vi "Lesson1 - Producer-Consumer Architecture and Queues.vi"() -> ()   [LabVIEW 2013]
uses:
  <vilib>/measure/NI_MABase.lvlib
panel:
  out "Waveform Graph":dbl[](graph)
  in  "Stop Button":bool
  out "Numeric 2":i32
  out "Numeric":i32
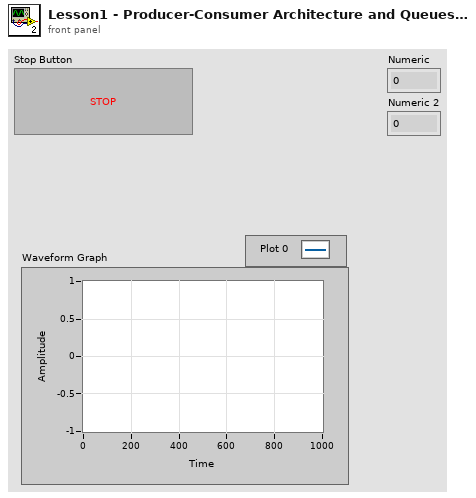
[diagram p1: front panel]
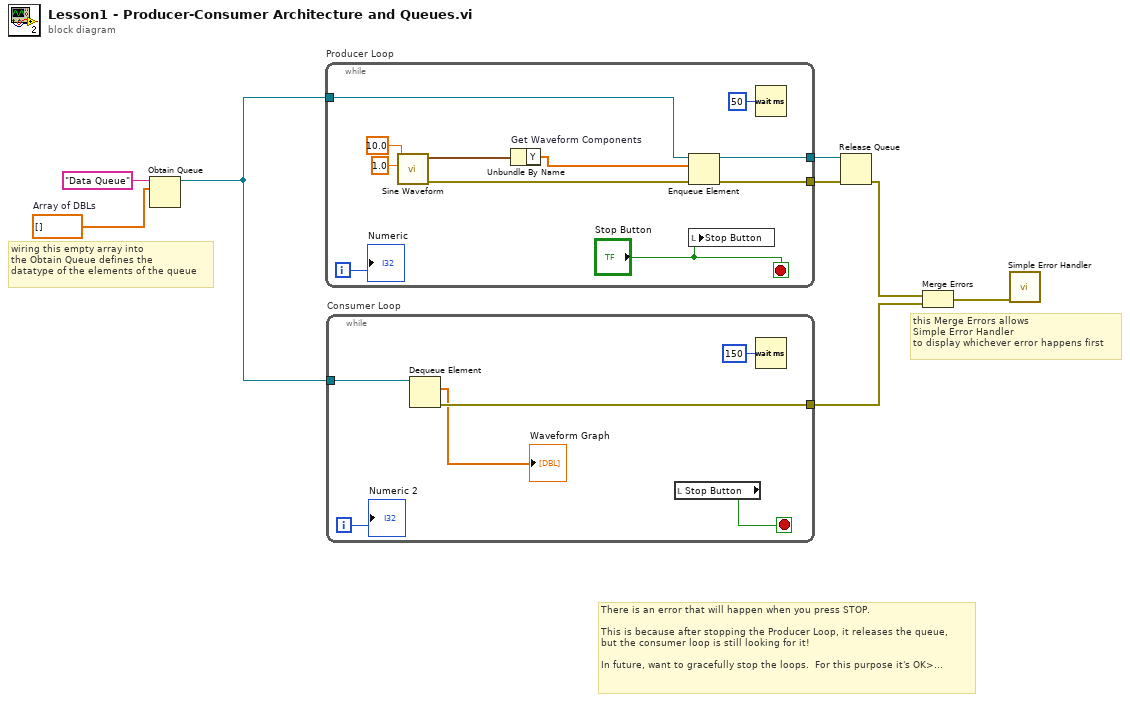
[diagram p0: block diagram]
diagram:
  w6 = dbl[] []  # Array of DBLs
  # "There is an error that will happen when you press STOP.\n\nThis is because after stopping the Producer Loop, it releases the queue,\nbut the consumer loop is still looking for it!\n\nIn future, want to gracefully stop the loops.  For this purpose it's OK>..."
  # "this Merge Errors allows \nSimple Error Handler \nto display whichever error happens first"
  # "wiring this empty array into\nthe Obtain Queue defines the\ndatatype of the elements of the queue"
  n1 = Obtain Queue(name (unnamed)="Data Queue", element data type=w6) -> (queue out=w7:refnum<queue>)  [unwired: 3 in, 2 out]
  n2 = while "Producer Loop" {
    tunnel: w7 -> [w12]
    tunnel: [w10] -> w5
    tunnel: [w9] -> w4
    i -> [w19]
    stop <- "Stop Button" stop-if-true
    n3 = call <vilib>:"Sine Waveform.vi"("amplitude"=1.0, "frequency"=10.0) -> ("error out"=w13:errorcluster, "signal out"=w14:waveform(dbl))  [unwired: 8 in]
    n4 = Unbundle By Name "Get Waveform Components"(w14) -> ("Y"=w11:dbl[])
    n5 = Enqueue Element(queue=w12, element=w11, error in (no error)=w13) -> (queue out=w10:refnum<queue>, error out=w9:errorcluster)  [unwired: 1 in, 1 out]
    n6 = local write "Stop Button"("Stop Button") -> ()
    n7 = Wait (ms)(milliseconds to wait=u32 50) -> ()  [unwired: 1 out]
    "Numeric" <- w19
  }
  n8 = while "Consumer Loop" {
    tunnel: w7 -> [w22]
    tunnel: [w21] -> w2
    i -> [w25]
    stop <- w24 stop-if-true
    n9 = Dequeue Element(queue=w22) -> (element=→"Waveform Graph":dbl[], error out=w21:errorcluster)  [unwired: 2 in, 2 out]
    n10 = local read "Stop Button"() -> (w24:bool)
    n11 = Wait (ms)(milliseconds to wait=u32 150) -> ()  [unwired: 1 out]
    "Numeric 2" <- w25
  }
  n12 = Release Queue(queue=w5, error in (no error)=w4) -> (error out=w3:errorcluster)  [unwired: 1 in, 2 out]
  n13 = Merge Errors "Merge Errors"(w3, w2) -> (w1:errorcluster)
  n14 = call <vilib>:"Simple Error Handler.vi"("error in (no error)"=w1) -> ()  [unwired: 4 in, 5 out]
